vi "AlgorithmCentralGoal - Copy.vi"(6 "MatchBallY":dbl, 7 "MatchBallX":dbl, 8 "D2 Y COM":dbl, 9 "D2 X COM":dbl, 10 "D1Y COM":dbl, 11 "D1 X COM":dbl) -> (0 "min x3":dbl, 1 "aS":dbl, 2 "min x2":dbl, 3 "aRW":dbl, 4 "min x":dbl, 5 "Theta LG,LW":dbl)   [LabVIEW 2014]
panel:
  out "xD2BotS":dbl
  out "xD2ComS":dbl
  out "xD1BotS":dbl
  out "xD1ComS":dbl
  out "xD2BotR":dbl
  out "xD2ComR":dbl
  out "xD1BotR":dbl
  out "xD1ComR":dbl
  out "D2 X Bot fit 2":dbl
  out "D2 X Com fit":dbl
  out "D1 X Bot fit":dbl
  out "D1 X Com fit":dbl
  # "LOGIC"
  # "Left Goal"
  # "STRAIGHT"
  # "Left wall"
  # "Right Wall"
  # "Straight"
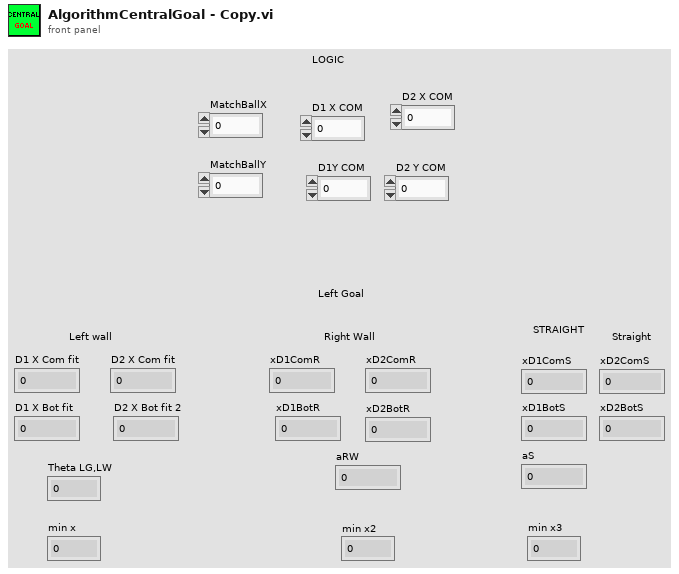
[diagram p1: front panel]
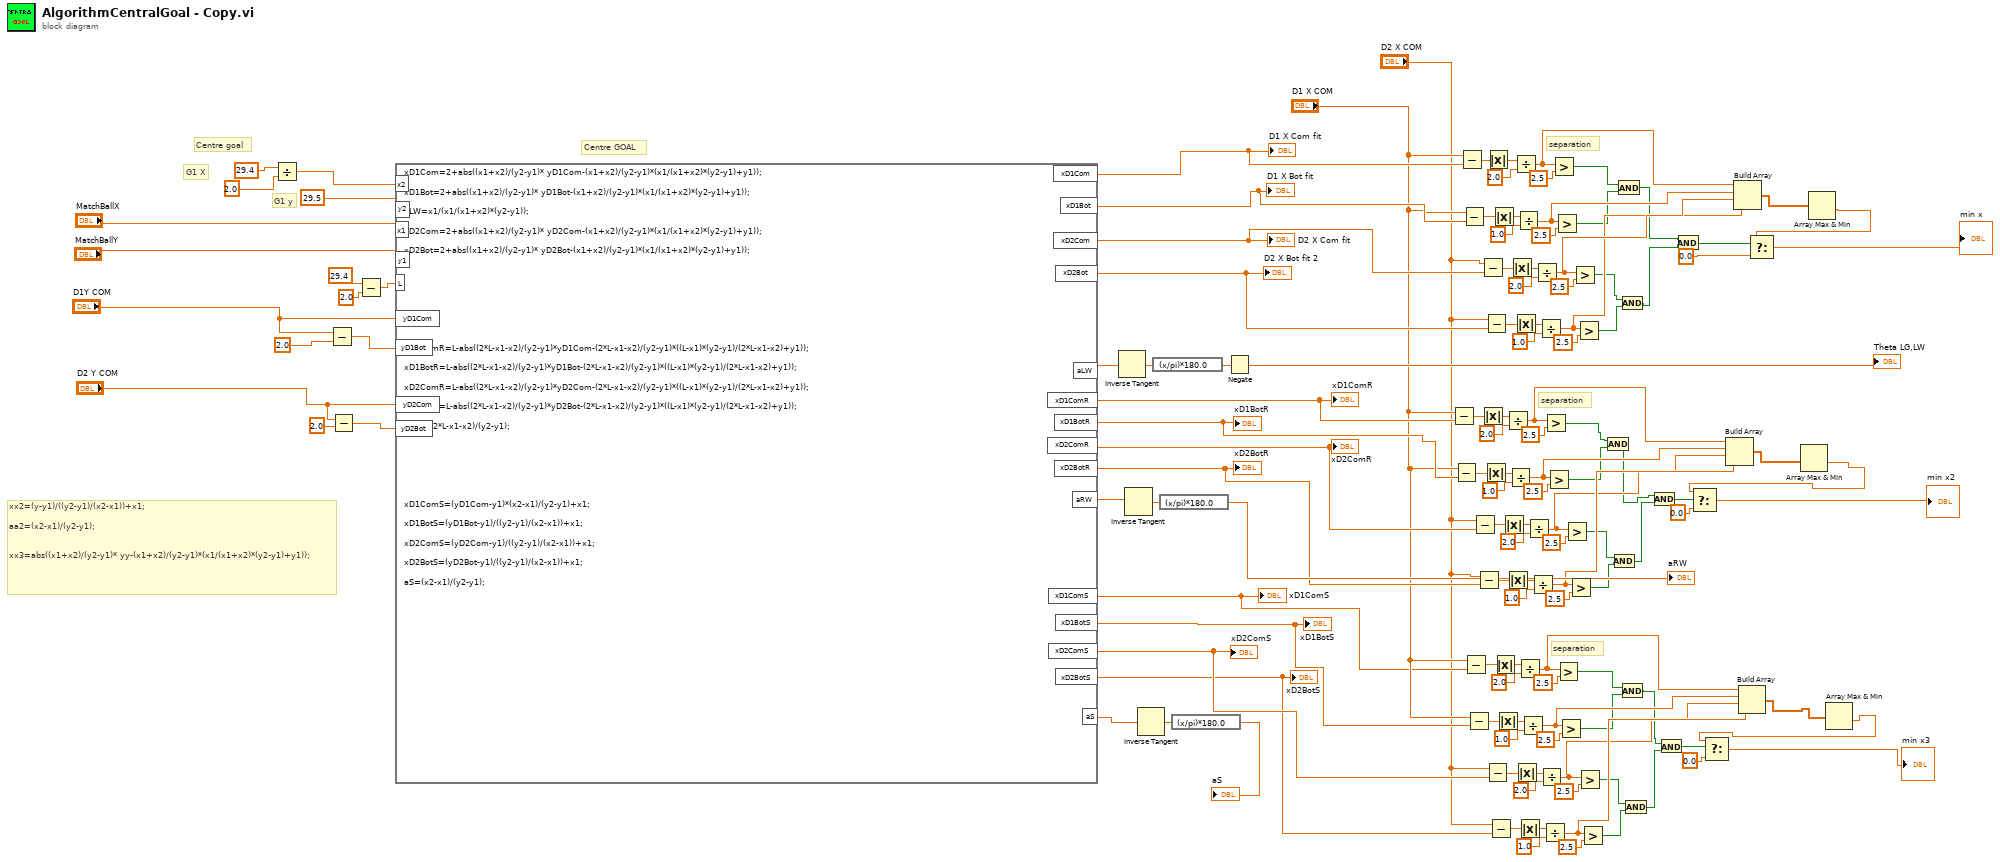
[diagram p0: block diagram]
diagram:
  # "separation"
  # "separation"
  # "separation"
  # "Centre GOAL"
  # "xx2=(y-y1)/((y2-y1)/(x2-x1))+x1;\n\naa2=(x2-x1)/(y2-y1);\n\n\nxx3=abs((x1+x2)/(y2-y1)* yy-(x1+x2)/(y2-y1)*(x1/(x1+x2)*(y2-y1)+y1));"
  # "Centre goal"
  # "G1 y"
  # "G1 X"
  n1 = Divide(x=29.4, y=2.0) -> (x/y=w5:dbl)
  n2 = Subtract(x="D1Y COM", y=2.0) -> (x-y=w125:dbl)
  n3 = Subtract(x="D2 Y COM", y=2.0) -> (x-y=w120:dbl)
  n4 = Subtract(x=29.4 ("input variable"), y=2.0) -> (x-y=w1:dbl)
  n5 = formula code="xD1Com=2+abs((x1+x2)/(y2-y1)* yD1Com-(x1+x2)/(y2-y1)*(x1/(x1+x2)*(y2-y1)+y1));\n\nxD1Bot=2+abs((x1+x2)/(y2-y1)* yD1Bot-(x1+x2)/(y2-y1)*(x1/(x1+x2)*(y2-y1)+y1));\n\naLW=x1/(x1/(x1+x2)*(y2-y1));\n\nxD2Com=2+abs((x1+x2)/(y2-y1)* yD2Com-(x1+x2)/(y2-y1)*(x1/(x1+x2)*(y2-y1)+y1));\n\nxD2Bot=2+abs((x1+x2)/(y2-y1)* yD2Bot-(x1+x2)/(y2-y1)*(x1/(x1+x2)*(y2-y1)+y1));\n\n\n\n\n\n\n\n\n\nxD1ComR=L-abs((2*L-x1-x2)/(y2-y1)*yD1Com-(2*L-x1-x2)/(y2-y1)*((L-x1)*(y2-y1)/(2*L-x1-x2)+y1));\n\nxD1BotR=L-abs((2*L-x1-x2)/(y2-y1)*yD1Bot-(2*L-x1-x2)/(y2-y1)*((L-x1)*(y2-y1)/(2*L-x1-x2)+y1));\n\nxD2ComR=L-abs((2*L-x1-x2)/(y2-y1)*yD2Com-(2*L-x1-x2)/(y2-y1)*((L-x1)*(y2-y1)/(2*L-x1-x2)+y1));\n\nxD2BotR=L-abs((2*L-x1-x2)/(y2-y1)*yD2Bot-(2*L-x1-x2)/(y2-y1)*((L-x1)*(y2-y1)/(2*L-x1-x2)+y1));\n\naRW=(2*L-x1-x2)/(y2-y1);\n\n\n\n\n\n\n\nxD1ComS=(yD1Com-y1)*(x2-x1)/(y2-y1)+x1;\n\nxD1BotS=(yD1Bot-y1)/((y2-y1)/(x2-x1))+x1;\n\nxD2ComS=(yD2Com-y1)/((y2-y1)/(x2-x1))+x1;\n\nxD2BotS=(yD2Bot-y1)/((y2-y1)/(x2-x1))+x1;\n\naS=(x2-x1)/(y2-y1);"("x1"="MatchBallX", "x2"=w5, "y2"=29.5, "y1"="MatchBallY", "yD1Com"="D1Y COM", "yD2Com"="D2 Y COM", "yD1Bot"=w125, "yD2Bot"=w120, "L"=w1) -> ("xD1Com"=w113:dbl, "aLW"=w128:dbl, "xD1Bot"=w99:dbl, "xD2Com"=w104:dbl, "xD2Bot"=w94:dbl, "xD1ComR"=w67:dbl, "xD1BotR"=w66:dbl, "xD2ComR"=w65:dbl, "xD2BotR"=w64:dbl, "aRW"=w118:dbl, "xD1ComS"=w41:dbl, "aS"=w114:dbl, "xD1BotS"=w40:dbl, "xD2BotS"=w38:dbl, "xD2ComS"=w39:dbl)
  "D1 X Com fit" <- w113
  "D1 X Bot fit" <- w99
  "D2 X Com fit" <- w104
  "D2 X Bot fit 2" <- w94
  "xD1ComR" <- w67
  "xD1BotR" <- w66
  "xD2ComR" <- w65
  "xD2BotR" <- w64
  "xD1ComS" <- w41
  "xD1BotS" <- w40
  "xD2ComS" <- w39
  "xD2BotS" <- w38
  n6 = Inverse Tangent(1:w128) -> (0:w129:dbl)
  n7 = Inverse Tangent(1:w118) -> (0:w119:dbl)
  n8 = Inverse Tangent(1:w114) -> (0:w115:dbl)
  n9 = expression code="(x/pi)*180.0" ("radians to degrees")(w129) -> (w126:dbl)
  n10 = expression code="(x/pi)*180.0" ("radians to degrees")(w119) -> (→"aRW":dbl)
  n11 = expression code="(x/pi)*180.0" ("radians to degrees")(w115) -> (→"aS":dbl)
  n12 = Negate(x=w126) -> (-x=→"Theta LG,LW":dbl)
  n13 = Subtract(x="D1 X COM", y=w67) -> (x-y=w68:dbl)
  n14 = Subtract(x="D1 X COM", y=w66) -> (x-y=w79:dbl)
  n15 = Subtract(x="D1 X COM", y=w113) -> (x-y=w112:dbl)
  n16 = Subtract(x="D1 X COM", y=w99) -> (x-y=w100:dbl)
  n17 = Subtract(x="D1 X COM", y=w41) -> (x-y=w43:dbl)
  n18 = Subtract(x="D1 X COM", y=w40) -> (x-y=w54:dbl)
  n19 = Subtract(x="D2 X COM", y=w65) -> (x-y=w75:dbl)
  n20 = Subtract(x="D2 X COM", y=w64) -> (x-y=w80:dbl)
  n21 = Subtract(x="D2 X COM", y=w104) -> (x-y=w105:dbl)
  n22 = Absolute Value(x=w68) -> (abs(x)=w69:dbl)
  n23 = Absolute Value(x=w79) -> (abs(x)=w78:dbl)
  n24 = Subtract(x="D2 X COM", y=w94) -> (x-y=w98:dbl)
  n25 = Subtract(x="D2 X COM", y=w39) -> (x-y=w50:dbl)
  n26 = Absolute Value(x=w112) -> (abs(x)=w111:dbl)
  n27 = Subtract(x="D2 X COM", y=w38) -> (x-y=w55:dbl)
  n28 = Absolute Value(x=w100) -> (abs(x)=w101:dbl)
  n29 = Absolute Value(x=w43) -> (abs(x)=w44:dbl)
  n30 = Absolute Value(x=w54) -> (abs(x)=w53:dbl)
  n31 = Absolute Value(x=w75) -> (abs(x)=w74:dbl)
  n32 = Divide(x=w69, y=2.0) -> (x/y=w85:dbl)
  n33 = Absolute Value(x=w80) -> (abs(x)=w81:dbl)
  n34 = Divide(x=w78, y=1.0) -> (x/y=w86:dbl)
  n35 = Absolute Value(x=w105) -> (abs(x)=w106:dbl)
  n36 = Divide(x=w111, y=2.0) -> (x/y=w92:dbl)
  n37 = Absolute Value(x=w98) -> (abs(x)=w97:dbl)
  n38 = Absolute Value(x=w50) -> (abs(x)=w49:dbl)
  n39 = Divide(x=w101, y=1.0) -> (x/y=w91:dbl)
  n40 = Divide(x=w44, y=2.0) -> (x/y=w60:dbl)
  n41 = Absolute Value(x=w55) -> (abs(x)=w56:dbl)
  n42 = Divide(x=w53, y=1.0) -> (x/y=w61:dbl)
  n43 = Divide(x=w74, y=2.0) -> (x/y=w87:dbl)
  n44 = Divide(x=w81, y=1.0) -> (x/y=w88:dbl)
  n45 = Divide(x=w106, y=2.0) -> (x/y=w90:dbl)
  n46 = Divide(x=w97, y=1.0) -> (x/y=w89:dbl)
  n47 = Divide(x=w49, y=2.0) -> (x/y=w62:dbl)
  n48 = Divide(x=w56, y=1.0) -> (x/y=w63:dbl)
  n49 = Greater?(x=w85, y=2.5) -> (0:w24:bool)
  n50 = Greater?(x=w86, y=2.5) -> (0:w23:bool)
  n51 = Greater?(x=w92, y=2.5) -> (0:w29:bool)
  n52 = Greater?(x=w91, y=2.5) -> (0:w28:bool)
  n53 = Greater?(x=w60, y=2.5) -> (0:w19:bool)
  n54 = Greater?(x=w61, y=2.5) -> (0:w18:bool)
  n55 = Greater?(x=w87, y=2.5) -> (0:w22:bool)
  n56 = Greater?(x=w88, y=2.5) -> (0:w21:bool)
  n57 = Greater?(x=w90, y=2.5) -> (0:w33:bool)
  n58 = Greater?(x=w89, y=2.5) -> (0:w32:bool)
  n59 = Greater?(x=w62, y=2.5) -> (0:w16:bool)
  n60 = Greater?(x=w63, y=2.5) -> (0:w15:bool)
  n61 = And(x=w24, y=w23) -> (x .and. y?=w25:bool)
  n62 = And(x=w22, y=w21) -> (x .and. y?=w20:bool)
  n63 = And(x=w29, y=w28) -> (x .and. y?=w27:bool)
  n64 = And(x=w33, y=w32) -> (x .and. y?=w30:bool)
  n65 = And(x=w19, y=w18) -> (x .and. y?=w17:bool)
  n66 = And(x=w16, y=w15) -> (x .and. y?=w14:bool)
  n67 = And(x=w25, y=w20) -> (x .and. y?=w26:bool)
  n68 = And(x=w17, y=w14) -> (x .and. y?=w13:bool)
  n69 = And(x=w27, y=w30) -> (x .and. y?=w31:bool)
  n70 = Build Array(w85, w86, w87, w88) -> (w10:dbl[])
  n71 = Build Array(w92, w91, w90, w89) -> (w12:dbl[])
  n72 = Build Array(w60, w61, w62, w63) -> (w8:dbl[])
  n73 = Array Max & Min(array=w10) -> (min value=w9:dbl)  [unwired: 3 out]
  n74 = Select(t=w9, s=w26, f=0.0 ("y")) -> (s? t:f=→"min x2":dbl)
  n75 = Array Max & Min(array=w12) -> (min value=w11:dbl)  [unwired: 3 out]
  n76 = Select(t=w11, s=w31, f=0.0 ("y")) -> (s? t:f=→"min x":dbl)
  n77 = Array Max & Min(array=w8) -> (min value=w7:dbl)  [unwired: 3 out]
  n78 = Select(t=w7, s=w13, f=0.0 ("y")) -> (s? t:f=→"min x3":dbl)
